vi "testAssertConnectorPanesMatchExpectedUnexpectedTerminalFound.vi"(8 "error in (no error)":errorcluster, 11 "TestCase in":refnum<class "VeriStandTestUtilitiesTests.lvclass">) -> (0 "error out":errorcluster, 3 "TestCase out":refnum<class "VeriStandTestUtilitiesTests.lvclass">)   [LabVIEW 2027, in "VeriStandTestUtilitiesTests.lvclass"]
uses:
  VeriStandTestUtilitiesTests.lvclass
  <vilib>/addons/_JKI Toolkits/VI Tester/TestCase.llb/TestCase.lvclass
  Source/VeriStandTestUtilities/VeriStandTestUtilities.lvlib
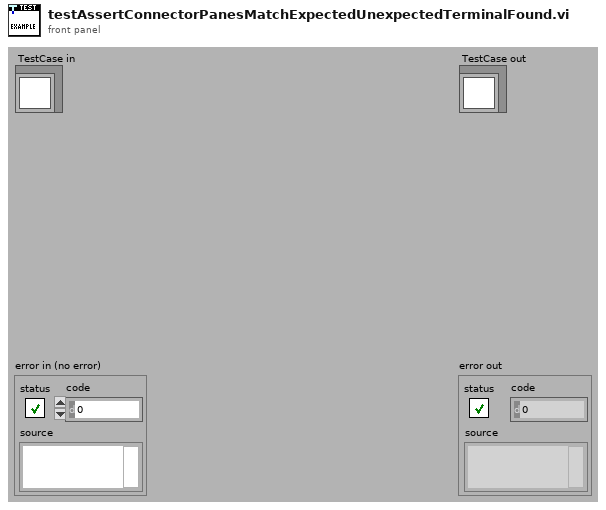
[diagram p1: front panel]
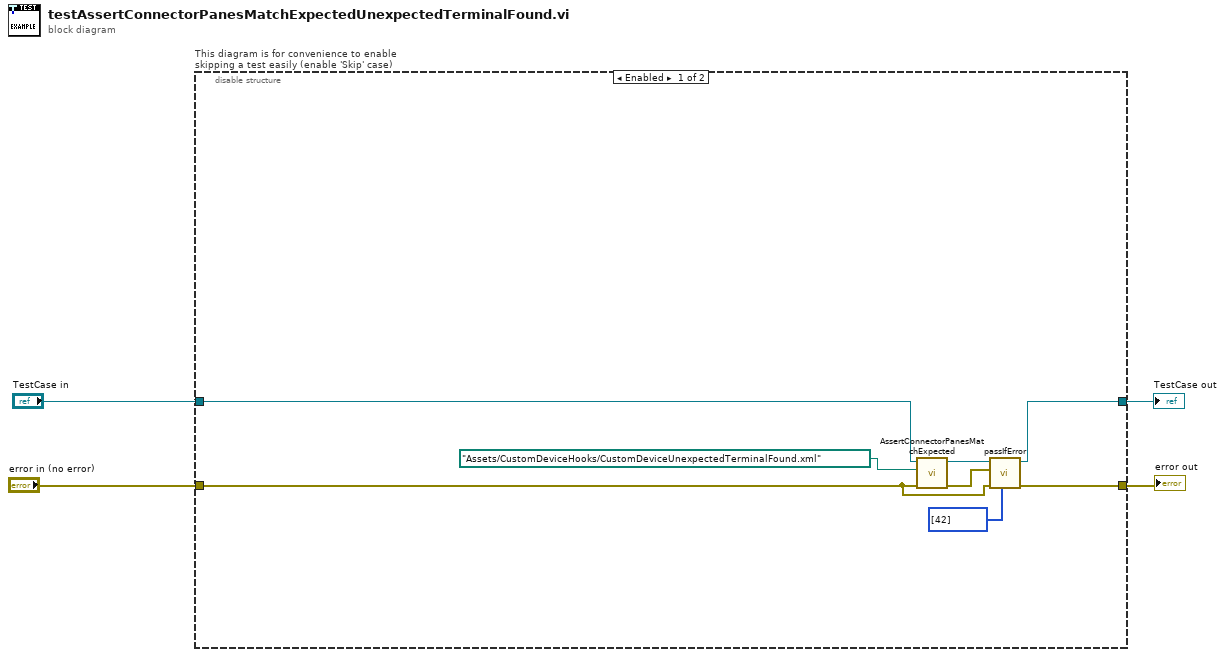
[diagram p0: block diagram]
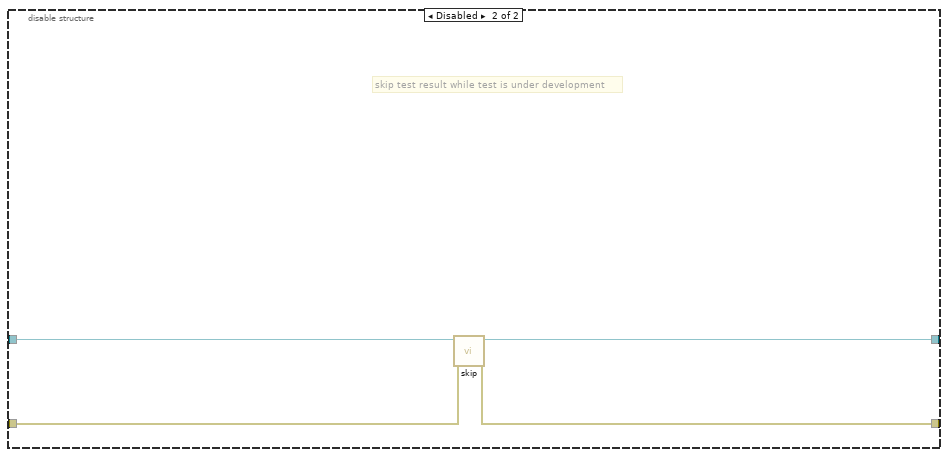
[diagram p2: hidden frame]
diagram:
  n1 = disable-structure "This diagram is for convenience to enable skipping a test easily (enable 'Skip' case)" shown="Enabled" {
    disable-tunnel: "TestCase in" -> [w10 w16]
    disable-tunnel: [w9 w14] -> w1
    disable-tunnel: [w11 w15] -> w3
    disable-tunnel: "error in (no error)" -> [w12 w13]
    frame Enabled {
      n2 = call "AssertConnectorPanesMatchExpected.vi"("error in (no error)"=w12, "custom device xml path"=path "Assets/CustomDeviceHooks/CustomDeviceUnexpectedTerminalFound.xml", "TestCase in"=w10) -> ("error out"=w7:errorcluster, "TestCase out"=w8:refnum<class "VeriStandTestUtilitiesTests.lvclass">)  [unwired: 7 in]
      n3 = call-dynamic "passIfError.vi"("passing error codes (default = any error code)"=i32[] [42], "error in (no error)"=w12, "error"=w7, "TestCase in"=w8) -> ("error out"=w11:errorcluster, "TestCase out"=w9:refnum<class "VeriStandTestUtilitiesTests.lvclass">)  [unwired: 6 in]
    }
    frame Disabled {
      # "skip test result while test is under development"
      n4 = call <vilib>:"skip.vi"("error in (no error)"=w13, "TestCase in"=w16) -> ("error out"=w15:errorcluster, "TestCase out"=w14:refnum<class "VeriStandTestUtilitiesTests.lvclass">)  [unwired: 8 in]
    }
  }
  "error out" <- w3
  "TestCase out" <- w1
